vi "Read ALR_ON_OFF_initialised.vi"(8 "error in (no error)":errorcluster, 11 "ALR in":T1) -> (0 "error out":errorcluster, 2 "initialised":u16, 3 "ALR out":T1)   [LabVIEW 2019, in "Alarms.lvlib"]
uses:
  Alarms.lvlib
  Ctl/Alarms.ctl
  Ctl/ALR_defs.ctl
  Ctl/ALRs_State.ctl
  Ctl/ALR_ON_OFF.ctl
  Ctl/ALR_Parameters.ctl
  Ctl/ALR code.ctl
  Ctl/ALR type.ctl
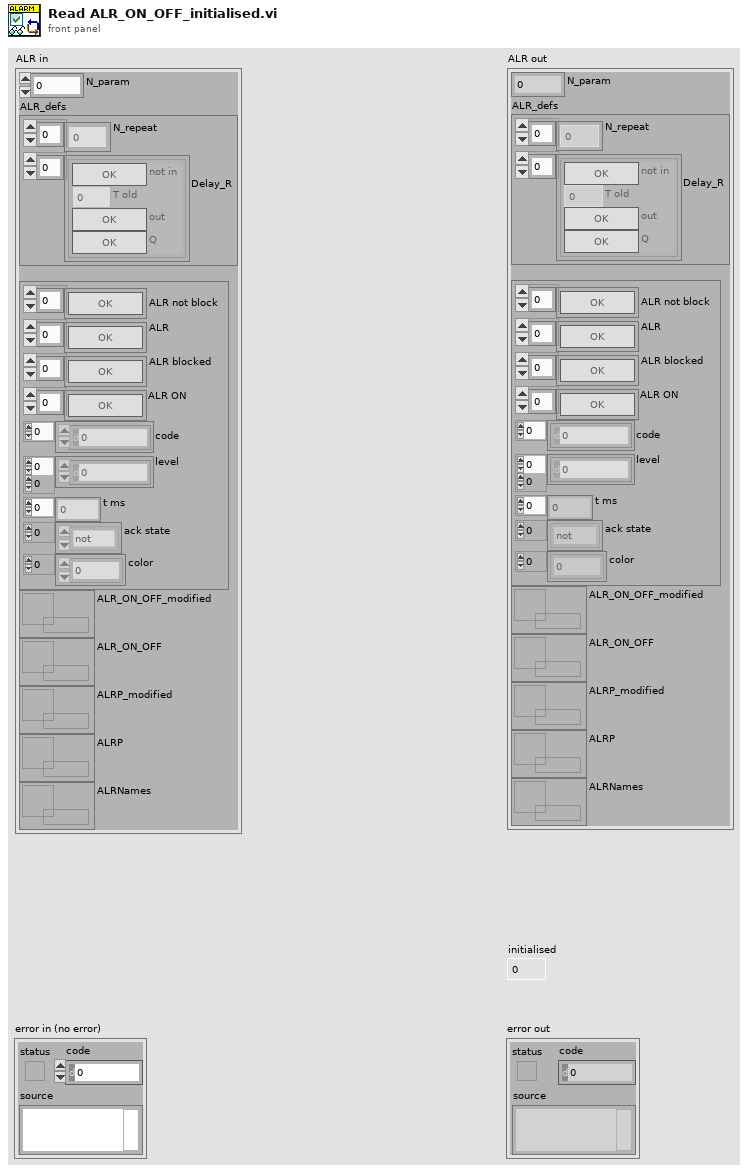
[diagram p1: front panel]
types:
  T1 = typedef "Alarms.lvlib/Alarms.ctl" = cluster{"N_param":i32, "ALR_defs":T2, "ALR_State":T3, "ALR_ON_OFF_modified":refnum<data-value>, "ALR_ON_OFF":refnum<data-value>, "ALRP_modified":refnum<data-value>, "ALRP":refnum<data-value>, "ALRNames":refnum<data-value>}
  T2 = typedef "Alarms.lvlib/ALR_defs.ctl" = cluster{"N_repeat":u32[], "Delay_R":cluster{"not in":bool, "T old":u32, "out":bool, "Q":bool}[]}
  T3 = typedef "Alarms.lvlib/ALRs_State.ctl" = cluster{"ALR not block":bool[], "ALR":bool[], "ALR blocked":bool[], "ALR ON":bool[], "code":i32[], "level":i32[][], "t ms":u32[], "ack state":enum32{"not", "tripped", "reset", "ack"}[], "color":u32[]}
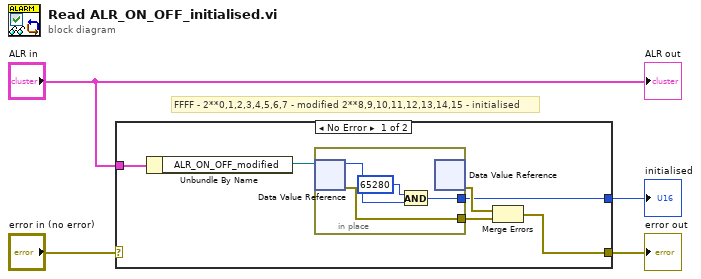
[diagram p0: block diagram]
diagram:
  # "FFFF - 2**0,1,2,3,4,5,6,7 - modified 2**8,9,10,11,12,13,14,15 - initialised"
  n1 = case shown="No Error" "error in (no error)" {
    selector: "error in (no error)" -> [_ w15]
    tunnel: [w7 w15] -> w1
    tunnel: "ALR in" -> [w6 _]
    tunnel: [w5 _] -> w2
    frame No Error {
      n2 = Unbundle By Name(w6) -> ("ALR_ON_OFF_modified"=w10:refnum<data-value>)
      n3 = in-place {
        in-place-border: [w14] -> w9
        in-place-border: [w11] -> w5
        n4 = in-place-dvr #1(w10) -> (w13:u16, w14:errorcluster)
        n5 = And(x=u16 65280 ("modified (0)"), y=w13) -> (x .and. y?=w11:u16)
        n6 = in-place-dvr #1() -> (w8:errorcluster)  [unwired: 1 in, 1 out]
      }
      n7 = Merge Errors(w8, w9) -> (w7:errorcluster)
    }
    frame Error {
    }
  }
  "error out" <- w1
  "initialised" <- w2
  "ALR out" <- "ALR in"
